vi "Control_MAIN.vi"() -> ()   [LabVIEW 2016]
uses:
  control vi/main/main/beamline selection.ctl
  control vi/main/main/upper subpanel selection.ctl
  control vi/save load/saveloadprev.ctl
  control vi/main/main/control_main_events.ctl
  cRIO code/SCA/controls/SCA commands.ctl
  control vi/main/main/main.lvlib
  control vi/save load/SaveLoad.lvlib
panel:
  in  "Clear Errors":bool
  in  "Preview-Save-Load":T1
  out "Abort error":errorcluster
  in  "change sample":bool
  in  "sample number":i16=1 min=1 max=64 step=1
  in  "pop? upper":bool
  out "Run-Time errors":errorcluster
  in  "Upper Panel":T2
  in  "pop? lower":bool
  in  "stop":bool
  in  "Lower Panel":T3
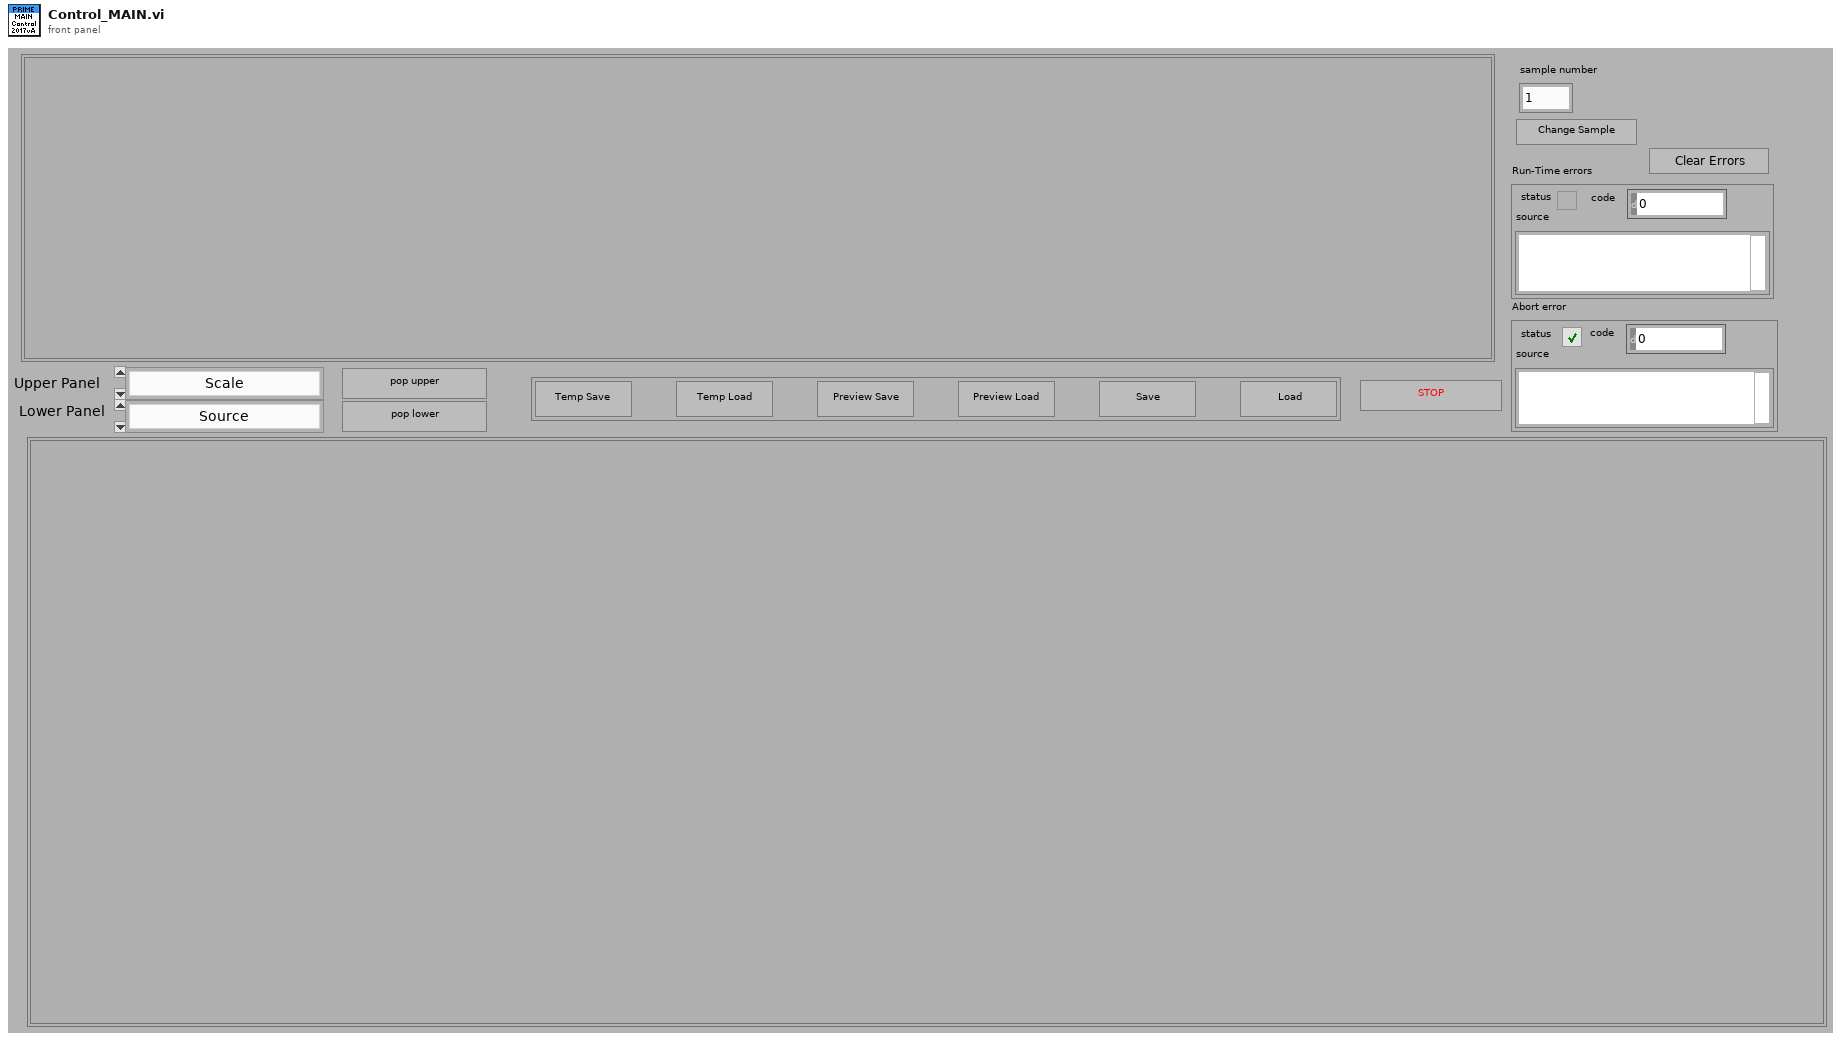
[diagram p1: front panel]
types:
  T1 = typedef "saveloadprev.ctl" = cluster{"Temp Save":bool, "Temp Load":bool, "Save":bool, "Load":bool, "Preview Save":bool, "Preview Load":bool}
  T2 = typedef "main.lvlib/upper subpanel selection.ctl" = enum16{"Scale", "Injector magnet", "Terminal Voltage", "Source BPM", "Beam Current", "Flat Top", "Scan Injector", "Scale - old"}
  T3 = typedef "main.lvlib/beamline selection.ctl" = enum16{"Source", "Low End", "High End", "Transmission", "R30", "R45"}
  T4 = typedef "control_main_events.ctl" = enum16{"Wait", "change lower panel", "change upper panel", "pop lower", "pop upper", "save-load", "Stop"}
  T5 = typedef "SCA commands.ctl" = enum16{"Wait", "Shutdown", "Retract insert rod", "Insert insert rod", "Retract retract rod", "Insert retract rod", "Retract sample rod", "Insert sample rod", "Open wheel GV", "Close wheel GV", "Open ion source GV", "Close ion source GV", "Pump out source", "Vent source", "Rotate wheel randomly", "Rotate wheel", "Start random sample change", "Start sample change"}
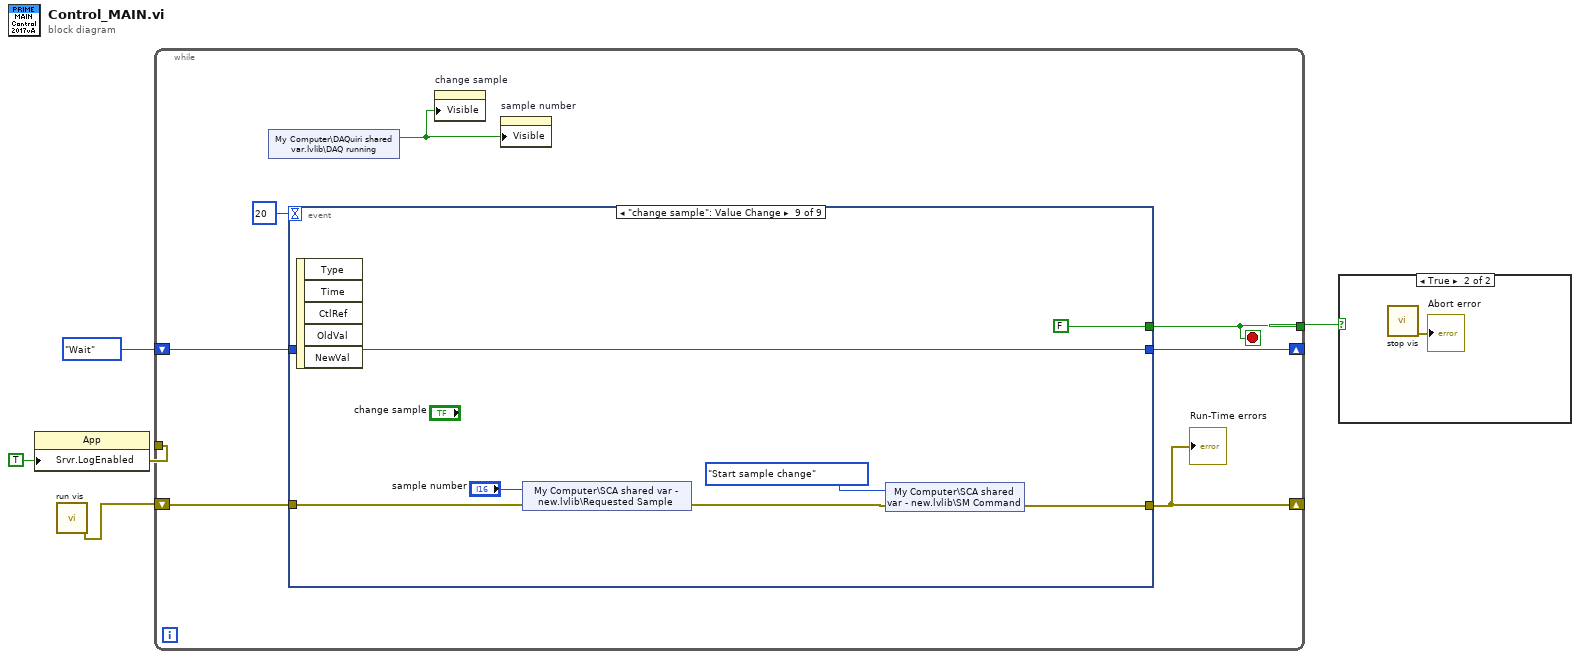
[diagram p0: block diagram]
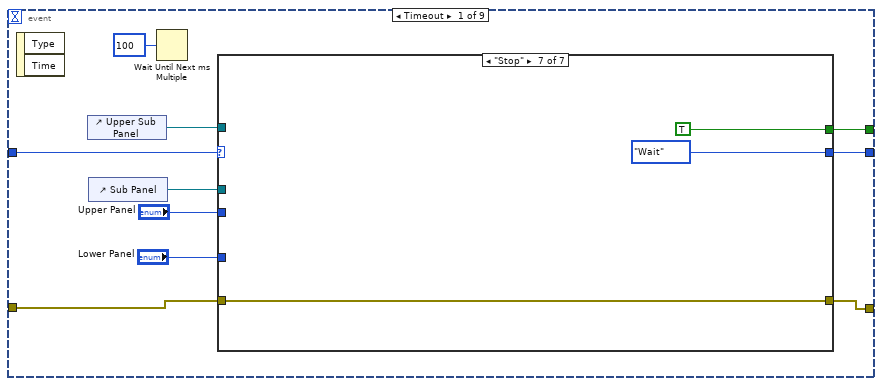
[diagram p3: hidden frame]
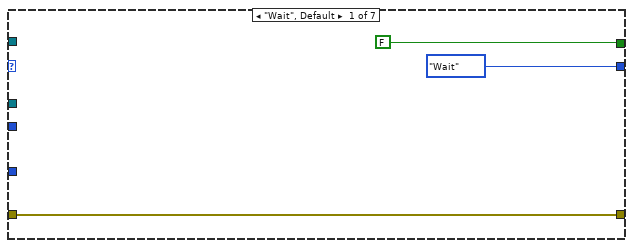
[diagram p4: hidden frame]
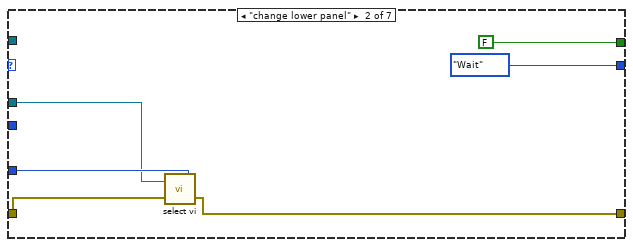
[diagram p5: hidden frame]
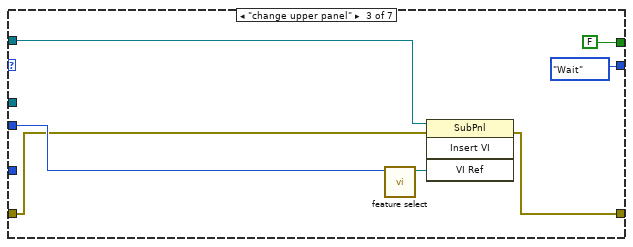
[diagram p6: hidden frame]
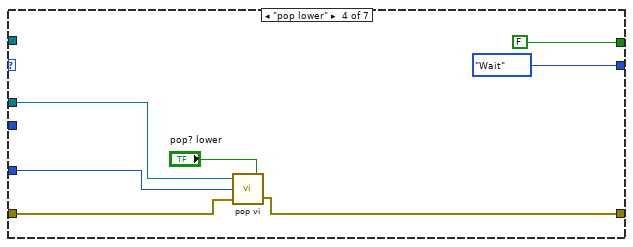
[diagram p7: hidden frame]
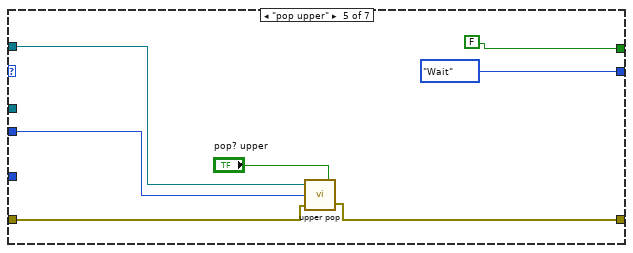
[diagram p8: hidden frame]
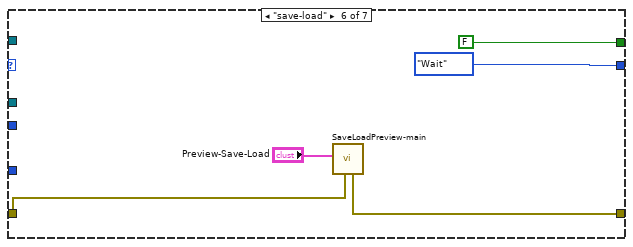
[diagram p9: hidden frame]
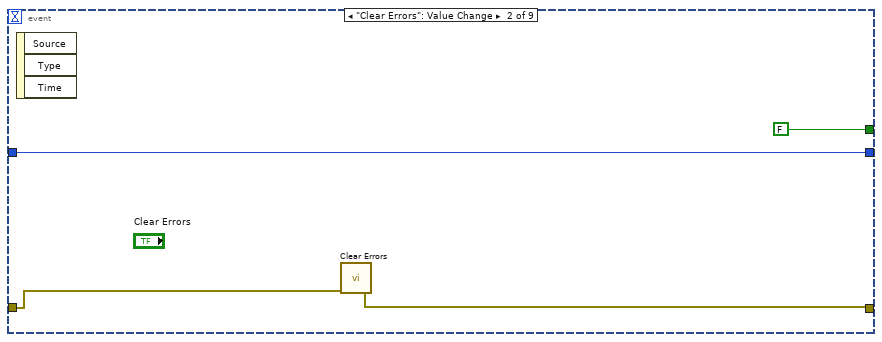
[diagram p10: hidden frame]
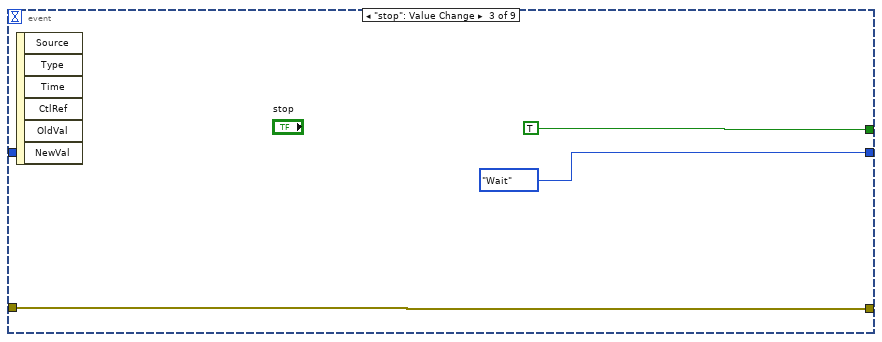
[diagram p11: hidden frame]
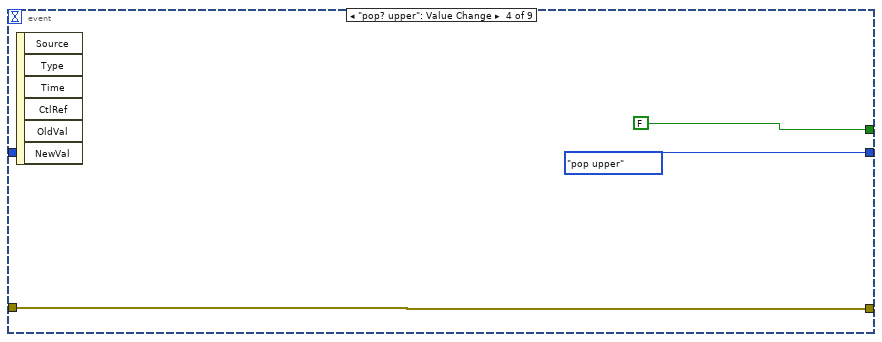
[diagram p12: hidden frame]
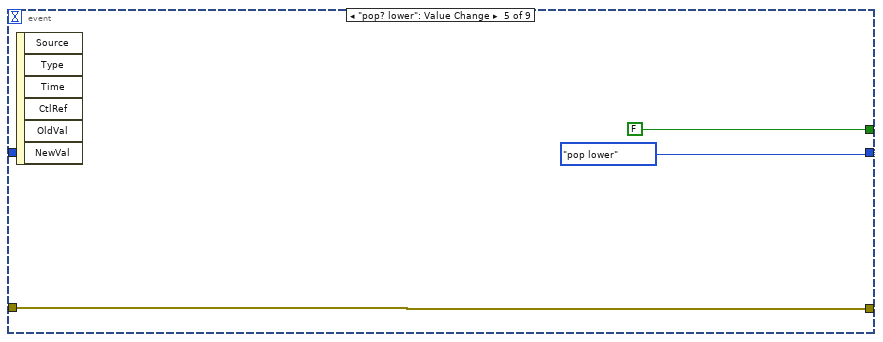
[diagram p13: hidden frame]
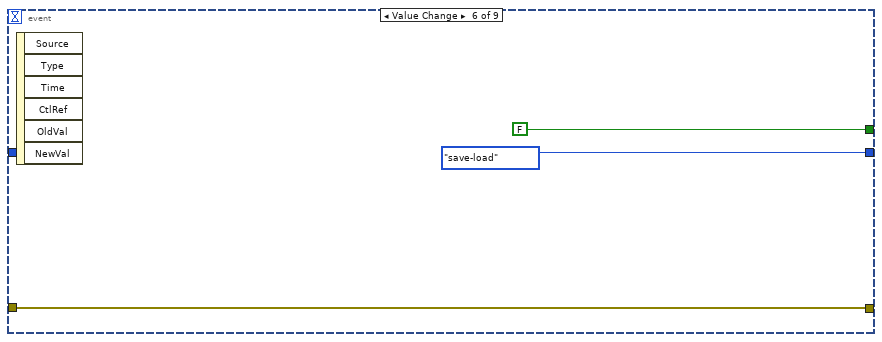
[diagram p14: hidden frame]
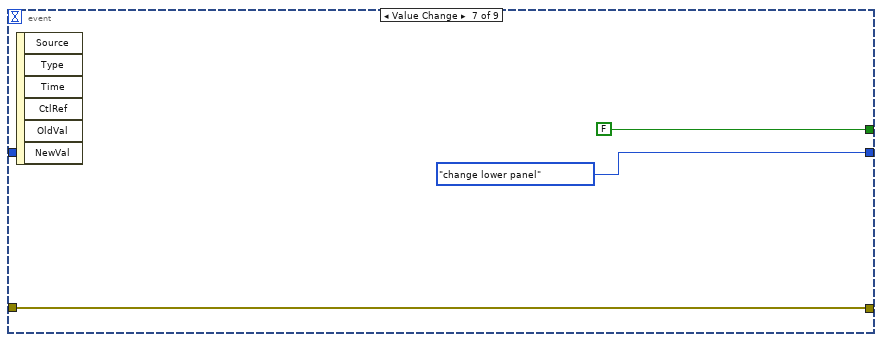
[diagram p15: hidden frame]
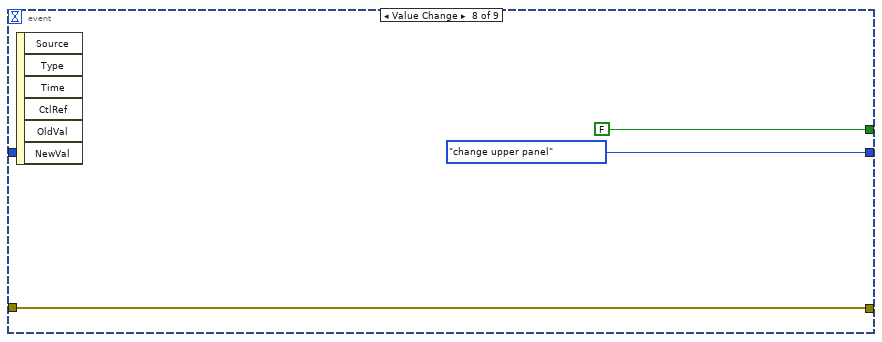
[diagram p16: hidden frame]
diagram:
  n1 = property class="App"("Srvr.LogEnabled"=TRUE ("Server:Logging Enabled")) -> (error out=w2:errorcluster)  [unwired: 2 in, 1 out]
  n2 = call "run vis.vi"() -> ("Tools and BL load error"=w1:errorcluster)  [unwired: 11 out]
  n3 = while {
    tunnel: [w10] -> w5
    shift-right: [w12] -> _
    shift-left: control_main_events."Wait" ("Ring") -> [w11]
    tunnel: w2 -> [_]
    shift-right: [w9] -> _
    shift-left: w1 -> [w8]
    stop <- w10 stop-if-true
    n4 = shared-variable "My Computer\\DAQuiri shared var.lvlib\\DAQ running"() -> (w6:bool)  [unwired: 1 in, 1 out]
    n5 = event shown="[8] \"change sample\": Value Change" {
      selector: _ -> [_ _ _ _ _ _ _ _ _]
      dyn-events: _ -> [_ _ _ _ _ _ _ _ _]
      timeout: 20 -> [_ _ _ _ _ _ _ _ _]
      tunnel: [w21 w63 control_main_events."Wait" ("Ring") control_main_events."pop upper" ("Ring") control_main_events."pop lower" ("Ring") control_main_events."save-load" ("Ring") control_main_events."change lower panel" ("Ring") control_main_events."change upper panel" ("Ring") w88] -> w12
      tunnel: w11 -> [w13 w63 _ _ _ _ _ _ w88]
      tunnel: [w20 FALSE ("stop") TRUE ("stop") FALSE ("stop") FALSE ("stop") FALSE ("stop") FALSE ("stop") FALSE ("stop") FALSE ("stop")] -> w10
      tunnel: [w15 w61 w65 w68 w71 w74 w77 w80 w85] -> w9
      tunnel: w8 -> [w14 w62 w65 w68 w71 w74 w77 w80 w84]
      event Timeout {
        n6 = event-data() -> ()  [unwired: 1 in, 2 out]
        n7 = control-ref of="Upper Sub Panel"() -> (w16:refnum<vi>)
        n8 = control-ref of="Sub Panel"() -> (w18:refnum<vi>)
        n9 = Wait Until Next ms Multiple(millisecond multiple=u32 100) -> ()  [unwired: 1 out]
        n10 = case shown="\"Stop\"" w13 {
          tunnel: [control_main_events."Wait" ("Ring") control_main_events."Wait" ("Ring") control_main_events."Wait" ("Ring") control_main_events."Wait" ("Ring") control_main_events."Wait" ("Ring") control_main_events."Wait" ("Ring") control_main_events."Wait" ("Ring")] -> w21
          tunnel: [FALSE ("stop") FALSE ("stop") FALSE ("stop") FALSE ("stop") FALSE ("stop") FALSE ("stop") TRUE ("stop")] -> w20
          tunnel: "Lower Panel" -> [_ w31 _ w43 _ _ _]
          tunnel: w18 -> [_ w30 _ w44 _ _ _]
          tunnel: "Upper Panel" -> [_ _ w36 _ w47 _ _]
          tunnel: w16 -> [_ _ w35 _ w48 _ _]
          tunnel: [w25 w28 w34 w41 w51 w53 w58] -> w15
          tunnel: w14 -> [w25 w27 w32 w40 w50 w56 w58]
          frame "Wait", Default {
          }
          frame "change lower panel" {
            n11 = call "select vi.vi"("Beamline Section"=w31, "error in (no error)"=w27, "reference"=w30) -> ("error out"=w28:errorcluster)
          }
          frame "change upper panel" {
            n12 = call "feature select.vi"("Feature Selection"=w36) -> ("VI Refnum"=w33:refnum<vi>)  [unwired: 1 in, 7 out]
            n13 = invoke on="Invoke Node" class="SubPnl" method="Insert VI"(reference=w35, error in=w32, "VI Ref"=w33) -> (error out=w34:errorcluster)  [unwired: 1 in, 3 out]
          }
          frame "pop lower" {
            n14 = call "pop vi.vi"("pop vi"="pop? lower", "error in (no error)"=w40, "Beamline Section"=w43, "Sub Panel"=w44) -> ("error out"=w41:errorcluster)
          }
          frame "pop upper" {
            n15 = call "upper pop.vi"("pop vi"="pop? upper", "error in (no error)"=w50, "Feature Selection"=w47, "Sub Panel"=w48) -> ("error out"=w51:errorcluster)
          }
          frame "save-load" {
            n16 = call "SaveLoadPreview-main.vi"("error in"=w56, "Prev-Save-Load"="Preview-Save-Load") -> ("error out 3"=w53:errorcluster)  [unwired: 9 in]
          }
          frame "Stop" {
          }
        }
      }
      event "Clear Errors": Value Change {
        n17 = event-data() -> ()  [unwired: 1 in, 3 out]
        n18 = call <vilib>:"Clear Errors.vi"("error in (no error)"=w62) -> ("error out"=w61:errorcluster)  [unwired: 5 in, 1 out]
      }
      event "stop": Value Change {
        n19 = event-data() -> ()  [unwired: 1 in, 6 out]
      }
      event "pop? upper": Value Change {
        n20 = event-data() -> ()  [unwired: 1 in, 6 out]
      }
      event "pop? lower": Value Change {
        n21 = event-data() -> ()  [unwired: 1 in, 6 out]
      }
      event Value Change {
        n22 = event-data() -> ()  [unwired: 1 in, 6 out]
      }
      event Value Change {
        n23 = event-data() -> ()  [unwired: 1 in, 6 out]
      }
      event Value Change {
        n24 = event-data() -> ()  [unwired: 1 in, 6 out]
      }
      event "change sample": Value Change {
        n25 = event-data() -> ()  [unwired: 1 in, 5 out]
        n26 = shared-variable "My Computer\\SCA shared var - new.lvlib\\Requested Sample"("sample number", error in=w84) -> (error out=w83:errorcluster)
        n27 = shared-variable "My Computer\\SCA shared var - new.lvlib\\SM Command"(SCA_commands."Start sample change" ("SM Command"), error in=w83) -> (error out=w85:errorcluster)
      }
    }
    "Run-Time errors" <- w9
    n28 = property on="change sample" class="Bool"("Visible"=w6) -> ()  [unwired: 2 in, 2 out]
    n29 = property on="sample number" class="DigNum (strict)"("Visible"=w6) -> ()  [unwired: 2 in, 2 out]
  }
  n30 = case shown="True" w5 {
    frame False {
    }
    frame True {
      n31 = call "stop vis.vi"() -> ("Abort error"=→"Abort error":errorcluster)  [unwired: 11 out]
    }
  }
